vi "Start.vi"(8 "error in (no error)":errorcluster, 11 "Object ref in":T1) -> (0 "error out":errorcluster, 3 "Object ref out":T1)   [LabVIEW 2013, in "HardwareCharacterization.lvlib" / "HC-Main.lvclass"]
uses:
  HC-Main.lvclass
  Object-reference.ctl
  HC-Main.lvclass/HC-Main.ctl
  Application-status.ctl
  UI/Control-names.ctl
  Process1-actions.ctl
  Read Measurement type.vi
  Read UI.vi
  Read Status.vi
  UI/Set-control-enable-multiple.vi
  UI/HC-UI.lvclass
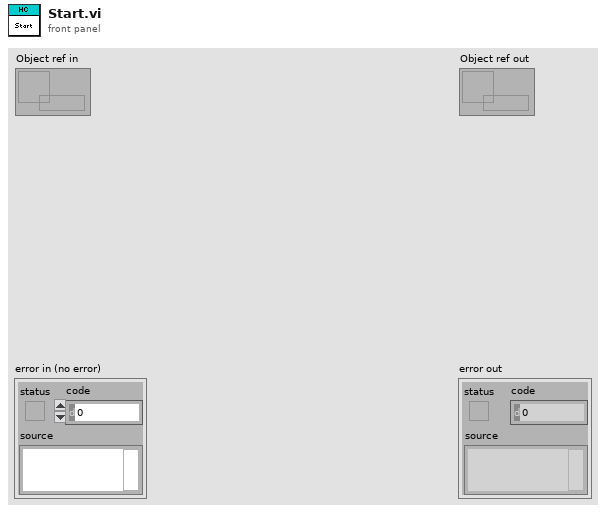
[diagram p1: front panel]
types:
  T1 = typedef "HardwareCharacterization.lvlib/HC-Main.lvclass/Object-reference.ctl" = refnum<data-value>
  T2 = typedef "HardwareCharacterization.lvlib/HC-Main.lvclass/Application-status.ctl" = enum16{"Idle", "Initialized", "Configured", "Activated", "Started", "Paused", "Stopped", "Reset", "Error", "Exited"}
  T3 = typedef "HardwareCharacterization.lvlib/HC-Main.lvclass/Process1-actions.ctl" = enum16{"Idle", "Activate", "Analyse scan file", "Convert SM1000positions", "Measure SM1000 timings", "Measure laser timings", "Stop", "Abort", "Exit"}
  T4 = typedef "HardwareCharacterization.lvlib/HC-UI.lvclass/Control-names.ctl" = enum16{"Help", "Status", "Load configuration", "Save configuration", "Activate", "Start", "Stop", "Options"}
  T5 = typedef "HardwareCharacterization.lvlib/HC-Main.lvclass/Measurement-types.ctl" = enum16{"Scan file analysis", "SM1000 position conversion", "SM1000 modulation timing", "Laser output response"}
  T6 = typedef "HardwareCharacterization.lvlib/HC-UI.lvclass/Panes-reference.ctl" = refnum<data-value>
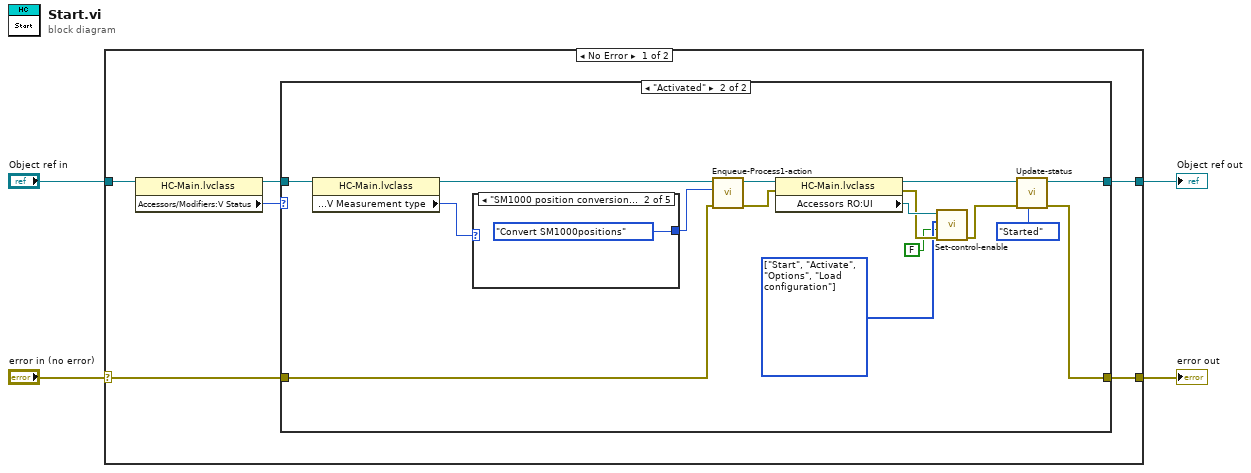
[diagram p0: block diagram]
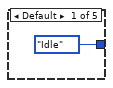
[diagram p3: hidden frame]
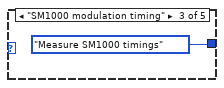
[diagram p4: hidden frame]
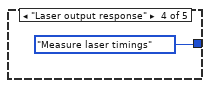
[diagram p5: hidden frame]
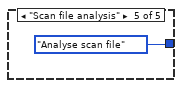
[diagram p6: hidden frame]
diagram:
  n1 = case shown="No Error" "error in (no error)" {
    selector: "error in (no error)" -> [w10 w35]
    tunnel: [w9 w35] -> w3
    tunnel: [w8 w34] -> w1
    tunnel: "Object ref in" -> [w7 w34]
    frame No Error {
      n2 = property class="HC-Main.lvclass"(reference=w7) -> (reference out=w6:T1, "Accessors/Modifiers:V Status"=w5:T2)  [unwired: 1 in, 1 out]
      n3 = case shown="\"Activated\"" w5 {
        tunnel: w6 -> [w12 w28]
        tunnel: w10 -> [w11 w27]
        tunnel: [w11 w25] -> w9
        tunnel: [w12 w24] -> w8
        frame Default {
        }
        frame "Activated" {
          w21 = T4[] [enum."Start", enum."Activate", enum."Options", enum."Load configuration"] items=["Help", "Status", "Load configuration", "Save configuration", "Activate", "Start", "Stop", "Options"] ("Control names")
          n4 = property class="HC-Main.lvclass"(reference=w28) -> (reference out=w14:T1, "Accessors/Modifiers:V Measurement type"=w13:T5)  [unwired: 1 in, 1 out]
          n5 = case shown="\"SM1000 position conversion\"" w13 {
            tunnel: [Process1-actions."Idle" ("Action") Process1-actions."Convert SM1000positions" ("Action") Process1-actions."Measure SM1000 timings" ("Action") Process1-actions."Measure laser timings" ("Action") Process1-actions."Analyse scan file" ("Action")] -> w17
            frame Default {
            }
            frame "SM1000 position conversion" {
            }
            frame "SM1000 modulation timing" {
            }
            frame "Laser output response" {
            }
            frame "Scan file analysis" {
            }
          }
          n6 = call "Enqueue-Process1-action.vi"("error in (no error)"=w27, "Action"=w17, "State queue in"=w14) -> ("error out"=w18:errorcluster, "State queue out"=w19:T1)  [unwired: 6 in, 1 out]
          n7 = property class="HC-Main.lvclass"(reference=w19, error in=w18) -> (reference out=w15:T1, error out=w22:errorcluster, "Accessors RO:UI"=w23:T6)
          n8 = call-poly "Set-control-enable.vi"("error in (no error)"=w22, "Enable?"=FALSE, "Control names"=w21, "Panes in"=w23) -> ("error out"=w16:errorcluster)  [unwired: 6 in, 1 out]
          n9 = call "Update-status.vi"("Status"=Application-status."Started", "error in (no error)"=w16, "Object ref in"=w15) -> ("error out"=w25:errorcluster, "Object ref out"=w24:T1)  [unwired: 7 in]
        }
      }
    }
    frame Error {
    }
  }
  "error out" <- w3
  "Object ref out" <- w1
